vi "h5_data.vi"(8 "error in (no error)":errorcluster, 11 "data":T1={"files"=[], "record"=FALSE, "save traces"=FALSE, "raw data"=[], "cursors"={"A"=0.0, "B"=0.0, "C"=0.0, "D"=0.0, "E"=0.0, "F"=0.0}, "analysis_result"={"var"=0.0, "w0"=0.0, "w1"=0.0, "a0"=0.0, "a1"=0.0, "a2"=0.0, "f"=0.0}, "analysis_pars"=[], "func"="a0 - a1"}) -> (0 "error out":errorcluster)   [LabVIEW 2017, in "tools.lvlib"]
uses:
  tools.lvlib
  data.ctl
  analysis/cursors.ctl
  analysis/analysis_result.ctl
  analysis/analysis_parameters.ctl
  <vilib>/UPVI/lvhdf5/dataset.llb/LVH5D Operation.ctl
  <vilib>/UPVI/lvhdf5/file.llb/LVH5F Operation.ctl
  <vilib>/UPVI/lvhdf5/dataset.llb/Simple OpenCreateReplace Dataset (Variant).vi
  <vilib>/Utility/VariantDataType/GetClusterInfo.vi
  <vilib>/Utility/VariantDataType/GetTypeInfo.vi
  <vilib>/UPVI/lvhdf5/attribute.llb/Write Multiple Attributes.vi
  <vilib>/UPVI/lvhdf5/attribute.llb/Simple H5Awrite (Variant).vi
  <vilib>/UPVI/lvhdf5/dataset.llb/H5Dwrite (Variant).vi
  <vilib>/UPVI/lvhdf5/dataset.llb/Append Element(s) to Dataset (Variant).vi
  <vilib>/UPVI/lvhdf5/dataset.llb/Simple OpenCreateReplace Dataset.xnode
  <vilib>/UPVI/lvhdf5/library.llb/HDF5 Ref.ctl
  <vilib>/UPVI/lvhdf5/attribute.llb/LVH5A Operation.ctl
  <vilib>/UPVI/lvhdf5/attribute.llb/LVH5 Write Attributes.xnode
  <vilib>/UPVI/lvhdf5/attribute.llb/Cluster to Attribute Array.xnode
  <vilib>/UPVI/lvhdf5/attribute.llb/Simple H5Awrite.xnode
  <vilib>/UPVI/lvhdf5/dataset.llb/H5Dwrite.xnode
  <vilib>/UPVI/lvhdf5/dataset.llb/Append Element(s) to Dataset.xnode
  <vilib>/Utility/VariantDataType/VariantType.lvlib
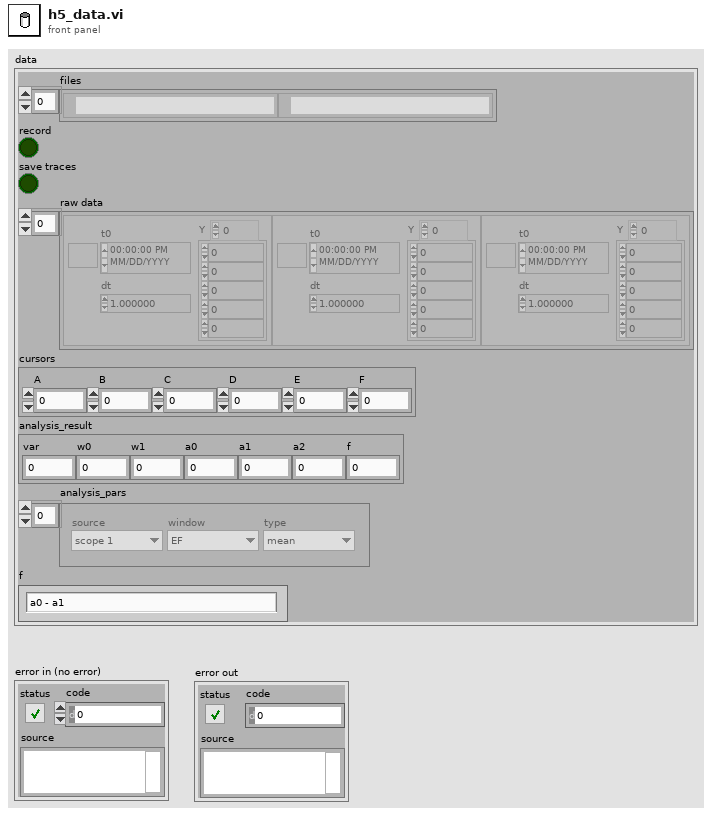
[diagram p1: front panel]
types:
  T1 = typedef "tools.lvlib/data.ctl" = cluster{"files":path[], "record":bool, "save traces":bool, "raw data":waveform(dbl)[], "cursors":T2, "analysis_result":T3, "analysis_pars":T4[], "func":string}
  T2 = typedef "tools.lvlib/cursors.ctl" = cluster{"A":dbl, "B":dbl, "C":dbl, "D":dbl, "E":dbl, "F":dbl}
  T3 = typedef "tools.lvlib/analysis_result.ctl" = cluster{"var":dbl, "w0":dbl, "w1":dbl, "a0":dbl, "a1":dbl, "a2":dbl, "f":dbl}
  T4 = typedef "tools.lvlib/analysis_parameters.ctl" = cluster{"source":enum16{"scope 0", "scope 1", "scope 2", "scope 3"}, "window":enum16{"AB", "CD", "EF"}, "type":enum16{"sum", "mean", "range"}}
  T5 = typedef "Semaphore RefNum" = refnum<k1>
  T6 = typedef "LVH5F Operation.ctl" = enum16{"open", "open or create", "create or replace", "create or replace (with confirmation)", "create", "open (read only)"}
  T7 = typedef "LVH5D Operation.ctl" = enum16{"open", "replace", "create", "open or create", "create or replace", "create or replace with confirmation"}
  T8 = typedef "HDF5 Ref.ctl" = refnum<k1>
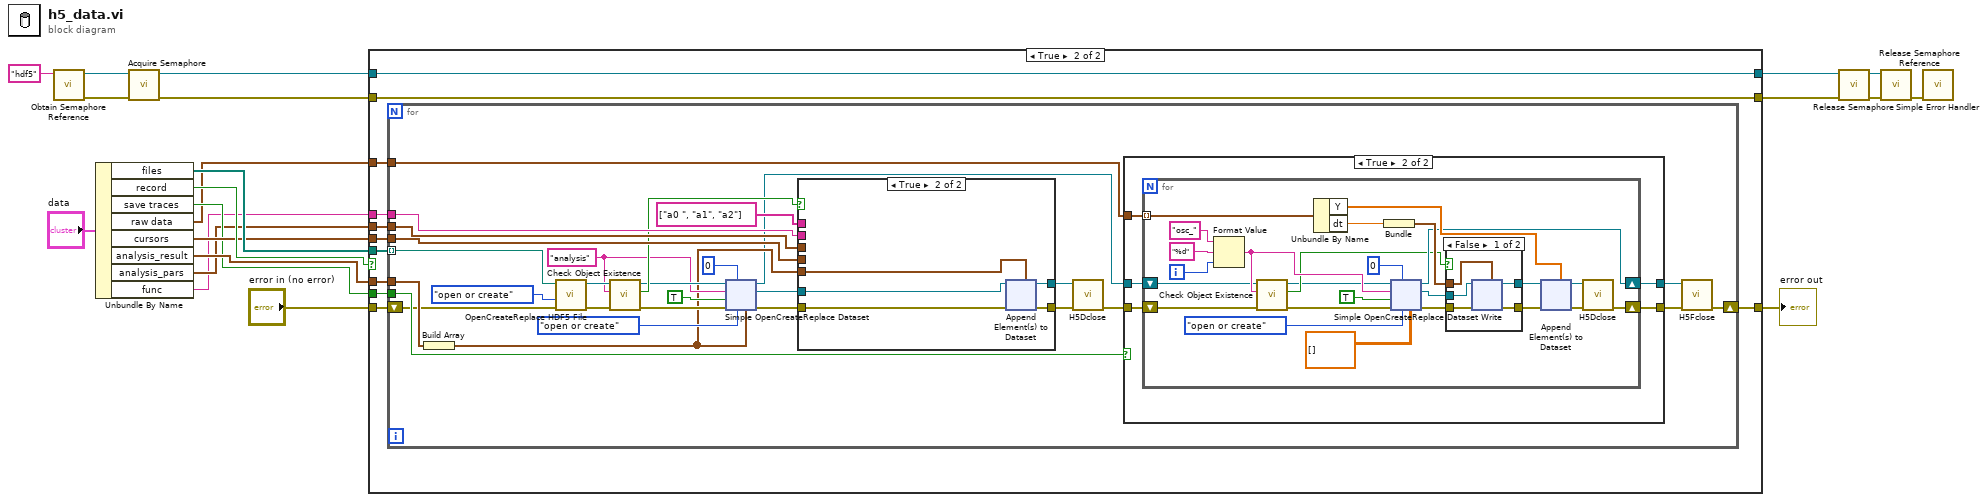
[diagram p0: block diagram]
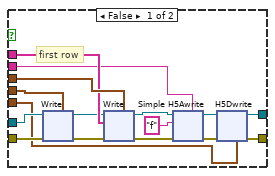
[diagram p5: hidden frame]
diagram:
  n1 = call <vilib>:"Obtain Semaphore Reference.vi"("name (unnamed)"="hdf5") -> ("error out"=w20:errorcluster, "semaphore"=w21:T5)  [unwired: 4 in, 1 out]
  n2 = Unbundle By Name("data") -> ("files"=w13:path[], "record"=w11:bool, "save traces"=w4:bool, "raw data"=w3:waveform(dbl)[], "cursors"=w6:T2, "analysis_result"=w5:T3, "analysis_pars"=w2:T4[], "func"=w1:string)
  n3 = call <vilib>:"Acquire Semaphore.vi"("error in (no error)"=w20, "semaphore"=w21) -> ("error out"=w10:errorcluster, "semaphore out"=w9:T5)  [unwired: 3 in, 1 out]
  n4 = case shown="True" w11 {
    tunnel: [w24 w35] -> w15
    tunnel: w13 -> [_ w34]
    tunnel: "error in (no error)" -> [w24 w33]
    tunnel: w10 -> [w23 w32]
    tunnel: w9 -> [w22 w31]
    tunnel: [w23 w32] -> w8
    tunnel: [w22 w31] -> w7
    tunnel: w6 -> [_ w30]
    tunnel: w5 -> [_ w29]
    tunnel: w4 -> [_ w28]
    tunnel: w3 -> [_ w27]
    tunnel: w2 -> [_ w26]
    tunnel: w1 -> [_ w25]
    frame False {
    }
    frame True {
      n5 = for {
        tunnel: w34 -> [w57] mode=indexing
        shift-right: [w43] -> w35
        shift-left: w33 -> [w56]
        tunnel: w30 -> [w64]
        tunnel: w29 -> [w63]
        tunnel: w28 -> [w62]
        tunnel: w27 -> [w61]
        tunnel: w26 -> [w59]
        tunnel: w25 -> [w58]
        w45 = "analysis" ("Dataset Path")
        n6 = Build Array(w63) -> (w42:T3[])
        n7 = call <vilib>:"OpenCreateReplace HDF5 File.vi"("error in (no error)"=w56, "function (open or create)"=LVH5F_Operation."open or create", "path"=w57) -> ("error out"=w54:errorcluster, "HDF5 Ref out"=w53:T8)  [unwired: 5 in]
        n8 = call <vilib>:"Check Object Existence.vi"("error in (no error)"=w54, "name"=w45, "HDF5 Ref"=w53) -> ("error out"=w49:errorcluster, "Exists"=w52:bool, "HDF5 Ref out"=w48:T8)  [unwired: 4 in]
        n9 = xnode "Simple OpenCreateReplace Dataset"("Compression Level (0-disabled)"=0, "Dataset Path"=w45, "HDF5 Ref"=w48, "Unlimited  dataset (F)"=TRUE, "error in (no error)"=w49, "operation"=LVH5D_Operation."open or create", "Datatype and Dataspace"=w42) -> ("HDF5 Dataset Ref out"=w44:T8, "HDF5 Ref out"=w38:T8, "error out"=w50:errorcluster)  [unwired: 1 in]
        n10 = case shown="True" w52 {
          tunnel: w50 -> [w263 w529]
          tunnel: w64 -> [w261 _]
          tunnel: string[] ["a0 ", "a1", "a2"] ("Name(s)") -> [w259 _]
          tunnel: w59 -> [w260 _]
          tunnel: w58 -> [w255 _]
          tunnel: w44 -> [w262 w530]
          tunnel: w42 -> [w248 w526]
          tunnel: [w249 w527] -> w41
          tunnel: [w250 w528] -> w40
          frame False {
            # "first row"
            n11 = xnode "Write"("HDF5 Ref"=w262, "error in (no error)"=w263, "Value(s)"=w261) -> ("HDF5 Ref out"=w253:T8, "error out"=w254:errorcluster)  [unwired: 2 in]
            n12 = xnode "Write"("HDF5 Ref"=w253, "error in (no error)"=w254, "Name(s)"=w259, "Value(s)"=w260) -> ("HDF5 Ref out"=w257:T8, "error out"=w256:errorcluster)  [unwired: 1 in]
            n13 = xnode "Simple H5Awrite"("HDF5 Ref"=w257, "Name"="f", "error in (no error)"=w256, "Value"=w255) -> ("HDF5 Ref out"=w252:T8, "error out"=w251:errorcluster)  [unwired: 1 in]
            n14 = xnode "H5Dwrite"("HDF5 Dataset Ref"=w252, "error in (no error)"=w251, "Data"=w248) -> ("HDF5 Ref out"=w249:T8, "error out"=w250:errorcluster)  [unwired: 4 in]
          }
          frame True {
            n15 = xnode "Append Element(s) to Dataset"("HDF5 Dataset Ref"=w530, "error in (no error)"=w529, "Data Element(s)"=w526) -> ("HDF5 Dataset out"=w527:T8, "error out"=w528:errorcluster)  [unwired: 1 in, 2 out]
          }
        }
        n16 = call <vilib>:"H5Dclose.vi"("error in (no error)"=w40, "HDF5 Dataset Ref"=w41) -> ("error out"=w39:errorcluster)  [unwired: 7 in]
        n17 = case shown="True" w62 {
          tunnel: [w65 w68] -> w37
          tunnel: w39 -> [w66 w70]
          tunnel: [w66 w69] -> w36
          tunnel: w61 -> [_ w71]
          tunnel: w38 -> [w65 w67]
          frame False {
          }
          frame True {
            n18 = for {
              tunnel: w71 -> [w89] mode=indexing
              shift-right: [w90] -> w69
              shift-left: w70 -> [w77]
              shift-right: [w78] -> w68
              shift-left: w67 -> [w74]
              i -> [w96]
              n19 = Format Value(string ("")="osc_", format string="%d", value (0)=w96) -> (output string=w75:string)
              n20 = call <vilib>:"Check Object Existence.vi"("error in (no error)"=w77, "name"=w75, "HDF5 Ref"=w74) -> ("error out"=w76:errorcluster, "Exists"=w73:bool, "HDF5 Ref out"=w72:T8)  [unwired: 4 in]
              n21 = Unbundle By Name(w89) -> ("Y"=w81:dbl[], "dt"=w88:dbl)
              n22 = Bundle("dt"=w88) -> (w87:cluster{"dt":dbl})  [unwired: 1 in]
              n23 = xnode "Simple OpenCreateReplace Dataset"("Compression Level (0-disabled)"=0, "Dataset Path"=w75, "HDF5 Ref"=w72, "Unlimited  dataset (F)"=TRUE, "error in (no error)"=w76, "operation"=LVH5D_Operation."open or create", "Datatype and Dataspace"=dbl[][] []) -> ("HDF5 Dataset Ref out"=w84:T8, "HDF5 Ref out"=w78:T8, "error out"=w91:errorcluster)  [unwired: 1 in]
              n24 = case shown="False" w73 {
                tunnel: w84 -> [w119 w236]
                tunnel: w91 -> [w120 w235]
                tunnel: [w116 w235] -> w83
                tunnel: w87 -> [w118 _]
                tunnel: [w117 w236] -> w80
                frame False {
                  n25 = xnode "Write"("HDF5 Ref"=w119, "error in (no error)"=w120, "Value(s)"=w118) -> ("HDF5 Ref out"=w117:T8, "error out"=w116:errorcluster)  [unwired: 2 in]
                }
                frame True {
                }
              }
              n26 = xnode "Append Element(s) to Dataset"("HDF5 Dataset Ref"=w80, "error in (no error)"=w83, "Data Element(s)"=w81) -> ("HDF5 Dataset out"=w79:T8, "error out"=w82:errorcluster)  [unwired: 1 in, 2 out]
              n27 = call <vilib>:"H5Dclose.vi"("error in (no error)"=w82, "HDF5 Dataset Ref"=w79) -> ("error out"=w90:errorcluster)  [unwired: 7 in]
            }
          }
        }
        n28 = call <vilib>:"H5Fclose.vi"("error in (no error)"=w36, "HDF5 Ref"=w37) -> ("error out"=w43:errorcluster)  [unwired: 7 in]
      }
    }
  }
  "error out" <- w15
  n29 = call <vilib>:"Release Semaphore.vi"("error in (no error)"=w8, "semaphore"=w7) -> ("error out"=w18:errorcluster, "semaphore out"=w17:T5)  [unwired: 4 in]
  n30 = call <vilib>:"Release Semaphore Reference.vi"("error in (no error)"=w18, "semaphore"=w17) -> ("error out"=w16:errorcluster)  [unwired: 8 in, 1 out]
  n31 = call <vilib>:"Simple Error Handler.vi"("error in (no error)"=w16) -> ()  [unwired: 4 in, 5 out]
